vi "Set Mediator Name.vi"(8 "error in (no error)":errorcluster caption="错误输入（无错误）", 10 "中介者":refnum<queue>, 11 "同事（抽象）输入":refnum<class "Colleague.lvclass">) -> (0 "error out":errorcluster caption="错误输出", 3 "同事（抽象）输出":refnum<class "Colleague.lvclass">)   [LabVIEW 2011]
uses:
  Colleague.lvclass
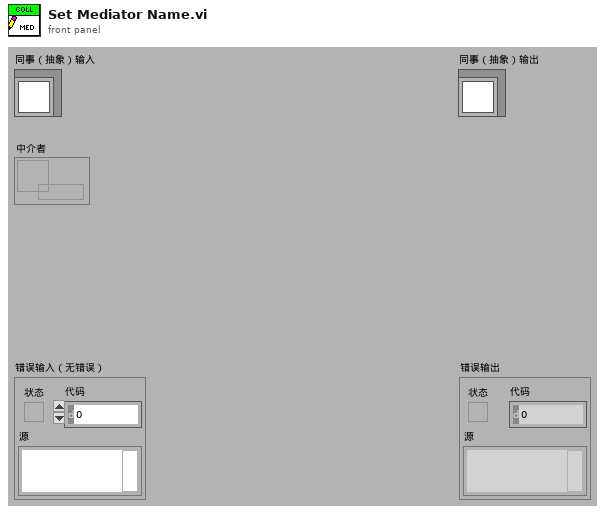
[diagram p1: front panel]
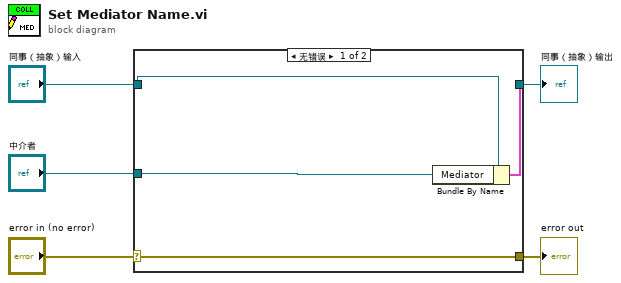
[diagram p0: block diagram]
diagram:
  n1 = case shown="无错误" "error in (no error)" {
    selector: "error in (no error)" -> [w9 w10]
    tunnel: [w9 w10] -> w4
    tunnel: [w7 w11] -> w2
    tunnel: "同事（抽象）输入" -> [w8 w11]
    tunnel: "中介者" -> [w6 _]
    frame No Error {
      n2 = Bundle By Name(cluster=w8, "Mediator"=w6) -> (w7:cluster{})
    }
    frame Error {
    }
  }
  "error out" <- w4
  "同事（抽象）输出" <- w2
